vi "Run Pre-Render Section.vi"(8 "Error In":errorcluster, 10 "Section In":refnum<class "Section.lvclass">, 11 "Context In":refnum<class "Compiler.lvclass">) -> (0 "Error Out":errorcluster, 2 "Section Out":refnum<class "Section.lvclass">, 3 "Context Out":refnum<class "Compiler.lvclass">)   [LabVIEW 2018, in "Toolkit.lvlib" / "Compiler.lvclass"]
uses:
  Compiler.lvclass
  Nodes/Section/Section.lvclass
  Compiler.lvclass/Compiler.ctl
  Hooks/Render/Section/Section.lvclass
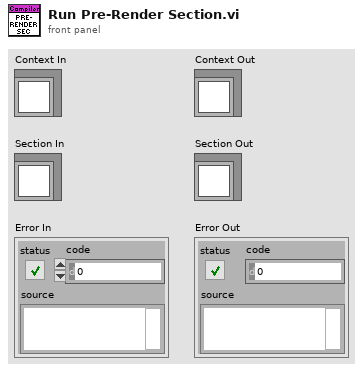
[diagram p1: front panel]
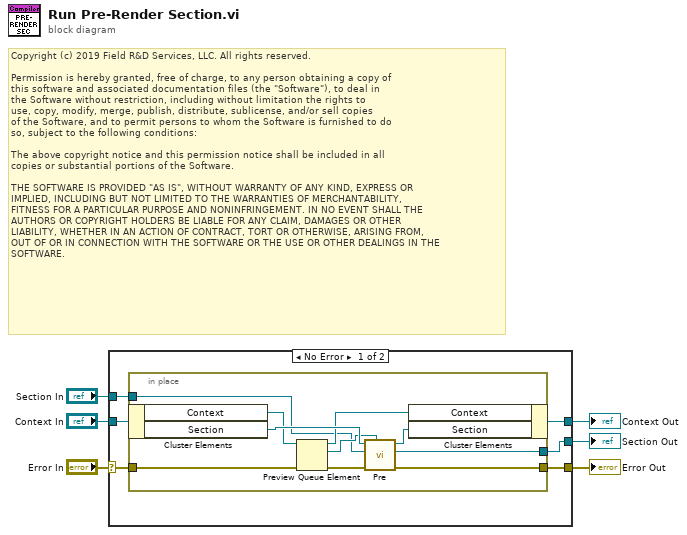
[diagram p0: block diagram]
diagram:
  # "Copyright (c) 2019 Field R&D Services, LLC. All rights reserved.\n\nPermission is hereby granted, free of charge, to any person obtaining a copy of\nthis software and associated documentation files (the \"Software\"), to deal in\nthe Software without restriction, including without limitation the rights to\nuse, copy, modify, merge, publish, distribute, sublicense, and/or sell copies\nof the Software, and to permit persons to whom the Software is furnished to do\nso, subject to the following conditions:\n\nThe above copyright notice and this permission notice shall be included in all\ncopies or substantial portions of the Software.\n\nTHE SOFTWARE IS PROVIDED \"AS IS\", WITHOUT WARRANTY OF ANY KIND, EXPRESS OR\nIMPLIED, INCLUDING BUT NOT LIMITED TO THE WARRANTIES OF MERCHANTABILITY,\nFITNESS FOR A PARTICULAR PURPOSE AND NONINFRINGEMENT. IN NO EVENT SHALL THE\nAUTHORS OR COPYRIGHT HOLDERS BE LIABLE FOR ANY CLAIM, DAMAGES OR OTHER\nLIABILITY, WHETHER IN AN ACTION OF CONTRACT, TORT OR OTHERWISE, ARISING FROM,\nOUT OF OR IN CONNECTION WITH THE SOFTWARE OR THE USE OR OTHER DEALINGS IN THE\nSOFTWARE."
  n1 = case shown="No Error" "Error In" {
    selector: "Error In" -> [w12 w24]
    tunnel: "Context In" -> [w9 w25]
    tunnel: [w11 w25] -> w4
    tunnel: [w10 w24] -> w3
    tunnel: [w8 w23] -> w1
    tunnel: "Section In" -> [w7 w23]
    frame No Error {
      n2 = in-place {
        in-place-border: w12 -> [w16]
        in-place-border: [w20] -> w10
        in-place-border: [w19] -> w8
        in-place-border: w7 -> [w13]
        n3 = in-place-cluster #1(w9) -> ("Context"=w18:refnum<queue>, "Section"=w22:refnum<class "Section.lvclass">)
        n4 = Preview Queue Element(queue=w18, error in (no error)=w16) -> (queue out=w17:refnum<queue>, element=w14:refnum<class "Datum.lvclass">, error out=w15:errorcluster)  [unwired: 1 in, 1 out]
        n5 = call-dynamic "Pre.vi"("Datum"=w14, "Error In"=w15, "Section In"=w13, "Render Section In"=w22) -> ("Error Out"=w20:errorcluster, "Section Out"=w19:refnum<class "Section.lvclass">, "Render Section Out"=w21:refnum<class "Section.lvclass">)  [unwired: 5 in]
        n6 = in-place-cluster #1("Context"=w17, "Section"=w21) -> (w11:refnum<class "Compiler.lvclass">)
      }
    }
    frame Error {
    }
  }
  "Context Out" <- w4
  "Error Out" <- w3
  "Section Out" <- w1
